vi "Start Lock-In Channel.vi"(7 "instance":i32, 8 "error in":errorcluster, 10 "config":cluster{"config":T1, "record length":u32}, 11 "lia host in":refnum<class "LIA Host Interface RT.lvclass">) -> (0 "error out":errorcluster, 3 "lia host out":refnum<class "LIA Host Interface RT.lvclass">)   [LabVIEW 2018, in "LIA Host Interface RT.lvclass"]
uses:
  LIA Host Interface RT.lvclass
  host/Public/lock-in settings.ctl
  shared/Public/message.ctl
  shared/Lock-In Amplifier Example Shared.lvlib
  host/Lock-In Amplifier Example Host.lvlib
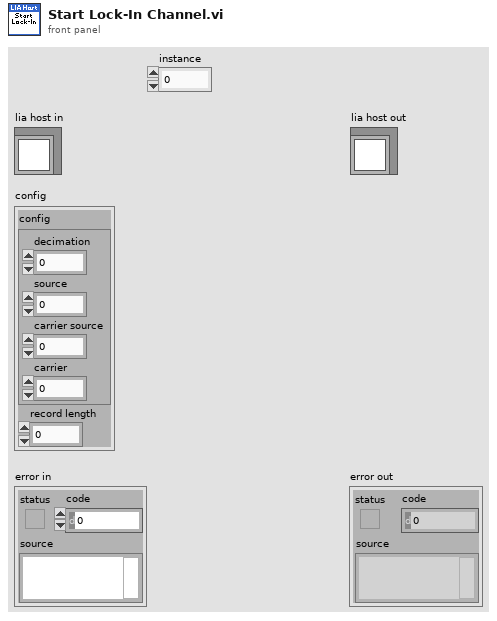
[diagram p1: front panel]
types:
  T1 = typedef "Lock-In Amplifier Example Host.lvlib/lock-in settings.ctl" = cluster{"decimation":i32, "source":i32, "carrier source":i32, "carrier":dbl}
  T2 = cluster{"instance":i32, "config":cluster{"config":T1, "record length":u32}}
  T3 = typedef "Lock-In Amplifier Example Shared.lvlib/message.ctl" = cluster{"command":u32, "payload":string}
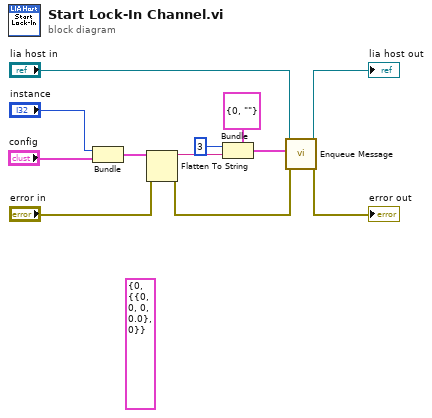
[diagram p0: block diagram]
diagram:
  (unwired) T2 {"instance"=0, "config"={"config"={"decimation"=0, "source"=0, "carrier source"=0, "carrier"=0.0}, "record length"=0}} ("output cluster")
  n1 = Bundle("instance"="instance", "config"="config") -> (w11:T2)  [unwired: 1 in]
  n2 = Flatten To String(anything=w11, error in (no error)="error in") -> (data string=w9:string, error out=w6:errorcluster)  [unwired: 2 in, 1 out]
  n3 = Bundle(cluster=T3 {"command"=0, "payload"=""} ("message"), "command"=u32 3, "payload"=w9) -> (w8:T3)
  n4 = call "Enqueue Message.vi"("error in"=w6, "command"=w8, "lia host in"="lia host in") -> ("error out"=→"error out":errorcluster, "lia host out"=→"lia host out":refnum<class "LIA Host Interface RT.lvclass">)  [unwired: 7 in]
